vi "Create Parameters.vi"(2 "error IO":errorcluster, 3 "parameters":T1[](array[typedef]), 4 "Parameters in":refnum<k7>, 5 "ADODB._Command":refnum<k7>) -> (0 "error out":errorcluster, 1 "Parameters out":refnum<k7>)   [LabVIEW 2011, in "Database Command.lvclass"]
uses:
  Database Command.lvclass
  <vilib>/addons/database/Auxilliary.llb/DB Tools Parameter Info.ctl
  <vilib>/addons/database/Auxilliary.llb/DB Tools DataTypes.ctl
  <vilib>/addons/database/Auxilliary.llb/DB Tools Parameter Dir.ctl
  <vilib>/addons/database/NI_Database_API.lvlib
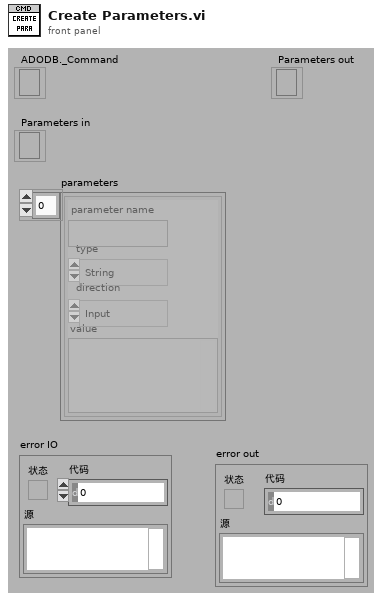
[diagram p1: front panel]
types:
  T1 = typedef "NI_Database_API.lvlib/DB Tools Parameter Info.ctl" = cluster{"parameter name":string, "type":T2, "direction":T3, "value":variant}
  T2 = typedef "NI_Database_API.lvlib/DB Tools DataTypes.ctl" = enum16{"String", "Long (I32)", "Single (SGL)", "Double (DBL)", "Date/Time", "Binary"}
  T3 = typedef "NI_Database_API.lvlib/DB Tools Parameter Dir.ctl" = enum32{"Input", "Output", "Input/Output", "Return Value"}
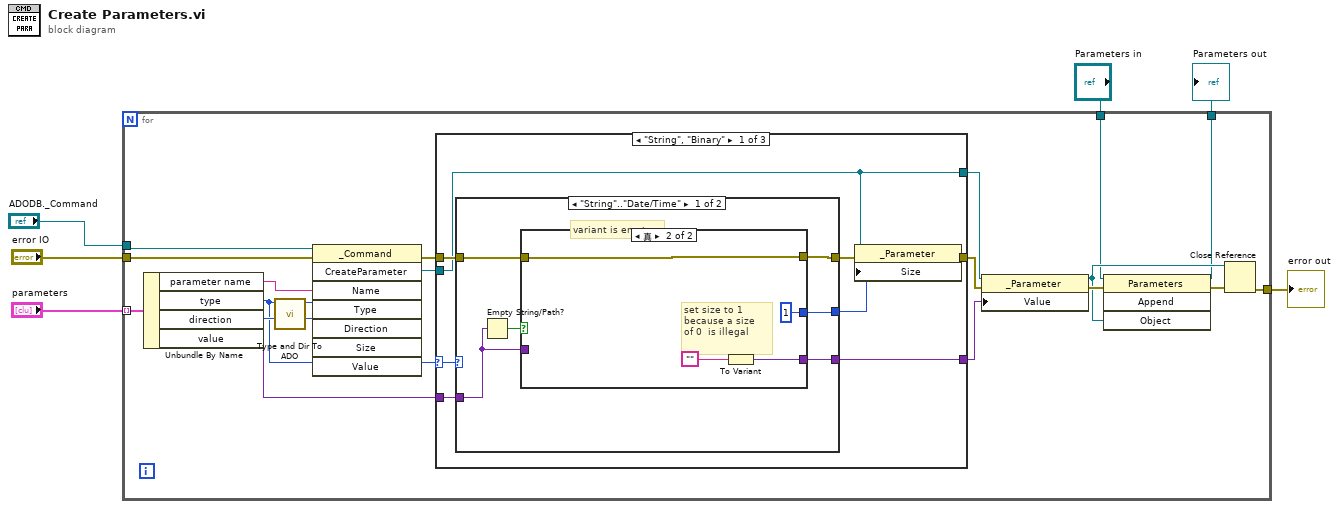
[diagram p0: block diagram]
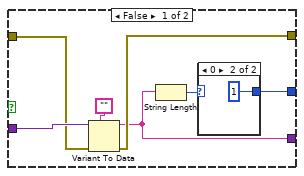
[diagram p2: hidden frame]
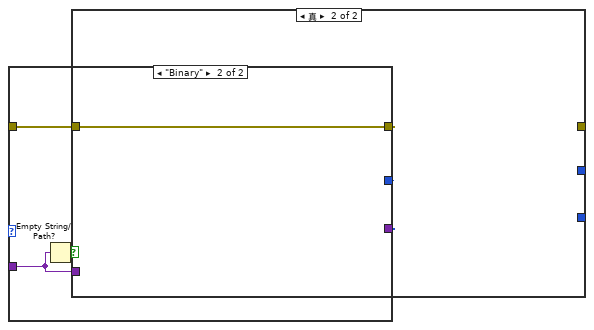
[diagram p4: hidden frame]
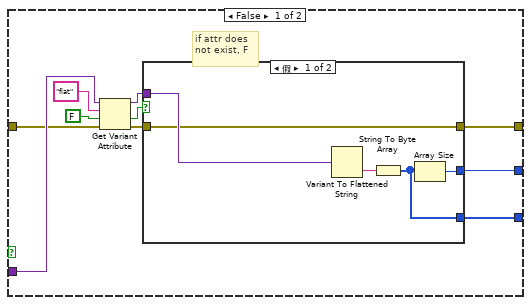
[diagram p5: hidden frame]
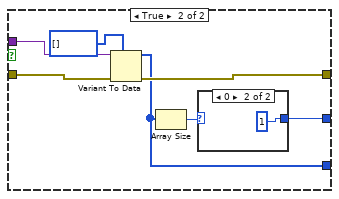
[diagram p6: hidden frame]
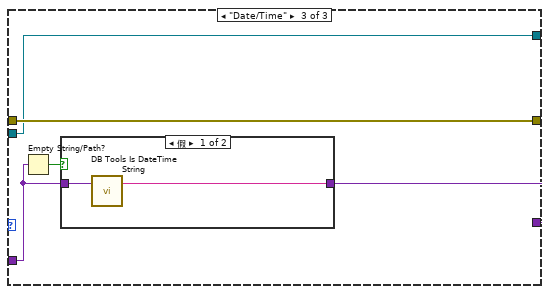
[diagram p9: hidden frame]
diagram:
  n1 = for {
    tunnel: "parameters" -> [w25] mode=indexing
    tunnel: "error IO" -> [w26]
    tunnel: [w7] -> w3
    tunnel: "ADODB._Command" -> [w16]
    tunnel: "Parameters in" -> [w9]
    tunnel: [w8] -> w6
    n2 = Unbundle By Name(w25) -> ("parameter name"=w21:string, "type"=w20:T2, "direction"=w24:T3, "value"=w19:variant)
    n3 = call "Type and Dir To ADO.vi"("direction"=w24, "data type"=w20) -> ("ADO direction"=w22:u16, "ADO type"=w23:u16)  [unwired: 8 in]
    n4 = invoke class="_Command" method="CreateParameter"(reference=w16, error in=w26, "Name"=w21, "Type"=w23, "Direction"=w22) -> (error out=w18:errorcluster, "CreateParameter"=w17:refnum<k7>)  [unwired: 3 in, 6 out]
    n5 = case shown="\"String\", \"Binary\"" w20 {
      selector: w20 -> [w32 _ _]
      tunnel: w19 -> [w31 w88 w91]
      tunnel: [w34 w89 w94] -> w15
      tunnel: w18 -> [w30 w89 w94]
      tunnel: [w28 w88 w93] -> w13
      tunnel: w17 -> [w27 w87 w90]
      tunnel: [w27 w87 w90] -> w14
      frame "String", "Binary" {
        n6 = case shown="\"String\"..\"Date/Time\"" w32 {
          tunnel: [w39 w58] -> w33
          tunnel: w31 -> [w38 w55]
          tunnel: w30 -> [w37 w54]
          tunnel: [w36 w57] -> w29
          tunnel: [w35 w56] -> w28
          frame "String".."Date/Time" {
            n7 = Empty String/Path?(string/path=w38) -> (empty?=w40:bool)
            n8 = case shown="真" w40 {
              tunnel: [w46 1] -> w39
              tunnel: w38 -> [w45 _]
              tunnel: w37 -> [w44 w52]
              tunnel: [w43 w52] -> w36
              tunnel: [w41 w50] -> w35
              frame False {
                n9 = Variant To Data(error in=w44, type="", Variant=w45) -> (data=w41:string, error out=w43:errorcluster)
                n10 = String Length(string=w41) -> (length=w47:i32)
                n11 = case shown="0" w47 {
                  selector: w47 -> [w48 _]
                  tunnel: [w48 1] -> w46
                  frame Default {
                  }
                  frame 0 {
                  }
                }
              }
              frame True {
                # "set size to 1 \nbecause a size \nof 0  is illegal"
                # "variant is empty"
                n12 = To Variant(anything="") -> (Variant=w50:variant)
              }
            }
          }
          frame "Binary" {
            n13 = Empty String/Path?(string/path=w55) -> (empty?=w59:bool)
            n14 = case shown="真" w59 {
              tunnel: [w68 1] -> w58
              tunnel: w54 -> [w65 w85]
              tunnel: [w69 w85] -> w57
              tunnel: [w67 u8[] [] ("Array Constant")] -> w56
              tunnel: w55 -> [w66 _]
              frame False {
                # "if attr does\nnot exist, F"
                n15 = Get Variant Attribute(Variant=w66, name="flat", default value (empty Variant)=FALSE, error in=w65) -> (duplicate Variant=w60:variant, value=w62:bool, error out=w61:errorcluster)  [unwired: 1 out]
                n16 = case shown="假" w62 {
                  tunnel: [w70 w81] -> w69
                  tunnel: [w71 w76] -> w68
                  tunnel: [w72 w79] -> w67
                  tunnel: w60 -> [w74 w78]
                  tunnel: w61 -> [w70 w77]
                  frame False {
                    n17 = Variant To Flattened String(Variant=w74) -> (data string=w73:string)  [unwired: 1 out]
                    n18 = String To Byte Array(string=w73) -> (unsigned byte array=w72:u8[])
                    n19 = Array Size(array=w72) -> (size(s)=w71:i32)
                  }
                  frame True {
                    n20 = Variant To Data(error in=w77, type=u8[] [] ("Array Constant"), Variant=w78) -> (data=w79:u8[], error out=w81:errorcluster)
                    n21 = Array Size(array=w79) -> (size(s)=w75:i32)
                    n22 = case shown="0" w75 {
                      selector: w75 -> [w82 _]
                      tunnel: [w82 1] -> w76
                      frame Default {
                      }
                      frame 0 {
                      }
                    }
                  }
                }
              }
              frame True {
                # "set size to 1 \nbecause\na size of 0\n is illegal"
                # "variant is empty"
              }
            }
          }
        }
        n23 = property class="_Parameter"(reference=w27, error in=w29, "Size"=w33) -> (error out=w34:errorcluster)  [unwired: 1 out]
      }
      frame "Long (I32)".."Double (DBL)" {
      }
      frame "Date/Time" {
        n24 = Empty String/Path?(string/path=w91) -> (empty?=w92:bool)
        n25 = case shown="假" w92 {
          tunnel: [w95 w97] -> w93
          tunnel: w91 -> [w96 w97]
          frame False {
            n26 = call <vilib>:"DB Tools Is DateTime String.vi"("string or date/time"=w96) -> ("data"=w95:string)  [unwired: 1 in, 1 out]
          }
          frame True {
          }
        }
      }
    }
    n27 = property class="_Parameter"(reference=w14, error in=w15, "Value"=w13) -> (reference out=w10:refnum<k7>, error out=w12:errorcluster)
    n28 = invoke class="Parameters" method="Append"(reference=w9, error in=w12, "Object"=w10) -> (reference out=w8:refnum<k7>, error out=w11:errorcluster)  [unwired: 1 in, 2 out]
    n29 = Close Reference(reference=w10, error in (no error)=w11) -> (error out=w7:errorcluster)
  }
  "Parameters out" <- w6
  "error out" <- w3
